vi "SA Cond - Insert Zeros.vi"(0 "wForm IN":waveform(dbl)[](array[waveform]), 5 "error in (no error)":errorcluster, 6 "Location":enum16{"In FRONT", "In BACK"}(ring), 7 "Selected Ch. Idx":i32, 9 "Nb Samples":i32, 10 "Anotate Signal Name":bool=TRUE) -> (14 "wForm OUT":waveform(dbl)[](array[waveform]), 19 "error out":errorcluster)   [LabVIEW 2022 SP3, in "GSwFormDSP.lvclass"]
uses:
  GSwFormDSP.lvclass
  Attribute List.ctl
  Attribute Options.ctl
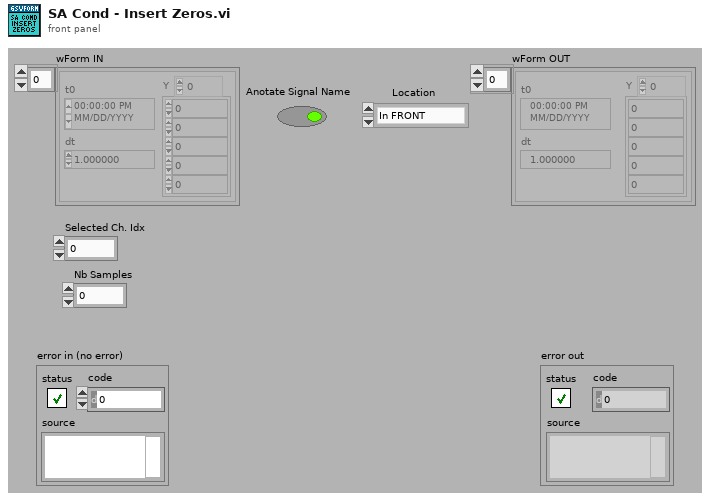
[diagram p1: front panel]
types:
  T1 = typedef "GSwFormDSP.lvclass/Attribute List.ctl" = string
  T2 = typedef "GSwFormDSP.lvclass/Attribute Options.ctl" = enum16{"Append to Attribute using \"( )\"", "Replace Attribute Value"}
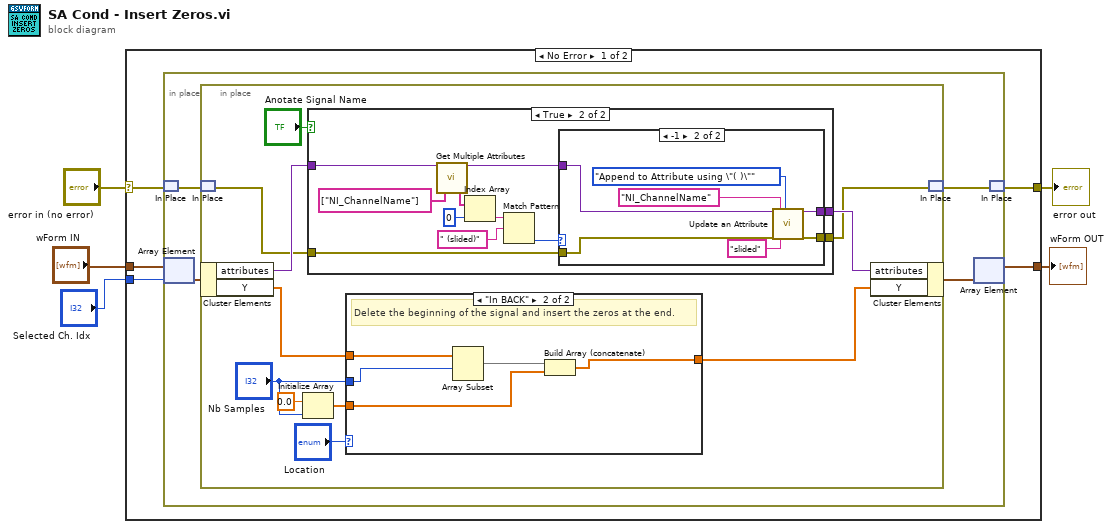
[diagram p0: block diagram]
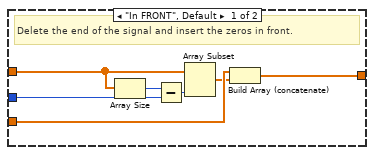
[diagram p2: hidden frame]
diagram:
  n1 = case shown="No Error" "error in (no error)" {
    selector: "error in (no error)" -> [w8 w61]
    tunnel: [w6 w61] -> w4
    tunnel: "wForm IN" -> [w10 w60]
    tunnel: "Selected Ch. Idx" -> [w9 _]
    tunnel: [w7 w60] -> w1
    frame No Error {
      n2 = in-place {
        n3 = in-place-match #1(w8) -> (w12:errorcluster)
        n4 = in-place-array #2(w10, w9) -> (w14:waveform(dbl))
        n5 = in-place {
          n6 = in-place-match #3(w12) -> (w18:errorcluster)
          n7 = in-place-cluster #4(w14) -> ("attributes"=w21:variant, "Y"=w16:dbl[])
          n8 = Initialize Array(0.0, "Nb Samples") -> (w23:dbl[])
          n9 = case shown="True" "Anotate Signal Name" {
            tunnel: w21 -> [w39 w50]
            tunnel: [w39 w42] -> w19
            tunnel: w18 -> [w38 w41]
            tunnel: [w38 w40] -> w17
            frame False {
            }
            frame True {
              n10 = call "Get Multiple Attributes.vi"("Attributes IN"=w50, "Attribute List"=T1[] ["NI_ChannelName"]) -> ("Values"=w48:string[], "Attributes OUT"=w43:variant)  [unwired: 16 in]
              n11 = Index Array(array=w48, index=0) -> (element=w45:string)
              n12 = Match Pattern(string=w45, regular expression=" (slided)" ("string")) -> (offset past match=w44:i32)  [unwired: 1 in, 3 out]
              n13 = case shown="-1" w44 {
                tunnel: w43 -> [w51 w59]
                tunnel: [w51 w56] -> w42
                tunnel: w41 -> [w52 w55]
                tunnel: [w52 w54] -> w40
                frame 0, Default {
                  # "The name has already been anotated"
                }
                frame -1 {
                  n14 = call "Update an Attribute.vi"("attributes in"=w59, "error in (no error)"=w55, "Attribute List"=T1 "NI_ChannelName", "Attribute Value"="slided" ("string"), "Attribute Option"=Attribute_Options."Append to Attribute using \"( )\"") -> ("attributes out"=w56:variant, "error out"=w54:errorcluster)  [unwired: 13 in]
                }
              }
            }
          }
          n15 = case shown="\"In BACK\"" "Location" {
            tunnel: "Nb Samples" -> [w31 w36]
            tunnel: w23 -> [w29 w34]
            tunnel: [w27 w33] -> w22
            tunnel: w16 -> [w26 w35]
            frame "In FRONT", Default {
              # "Delete the end of the signal and insert the zeros in front."
              n16 = Array Size(array=w26) -> (size(s)=w32:i32)
              n17 = Subtract(x=w32, y=w31) -> (x-y=w30:i32)
              n18 = Array Subset(array=w26, length=w30) -> (w28:dbl[])  [unwired: 1 in]
              n19 = Build Array (concatenate)(w29, w28) -> (w27:dbl[])
            }
            frame "In BACK" {
              # "Delete the beginning of the signal and insert the zeros at the end."
              n20 = Array Subset(array=w35, index=w36) -> (w37:dbl[])  [unwired: 1 in]
              n21 = Build Array (concatenate)(w37, w34) -> (w33:dbl[])
            }
          }
          n22 = in-place-cluster #4("attributes"=w19, "Y"=w22) -> (w13:waveform(dbl))
          n23 = in-place-match #3(w17) -> (w11:errorcluster)
        }
        n24 = in-place-array #2(w13) -> (w7:waveform(dbl)[])  [unwired: 1 out]
        n25 = in-place-match #1(w11) -> (w6:errorcluster)
      }
    }
    frame Error {
    }
  }
  "error out" <- w4
  "wForm OUT" <- w1
